vi "Update Zone.vi"(8 "error in (no error)":errorcluster, 9 "Zone Instance":refnum<class "Zone.lvclass">, 10 "Zone Name":string, 11 "TrafficMap in":refnum<class "TrafficMap.lvclass">) -> (0 "error out":errorcluster, 3 "TrafficMap out":refnum<class "TrafficMap.lvclass">)   [LabVIEW 2017, in "TrafficMap.lvclass"]
uses:
  TrafficMap.lvclass
  Zone/Zone.lvclass
  TrafficMap.lvclass/TrafficMap.ctl
  Zone/Zone.lvclass/Zone.ctl
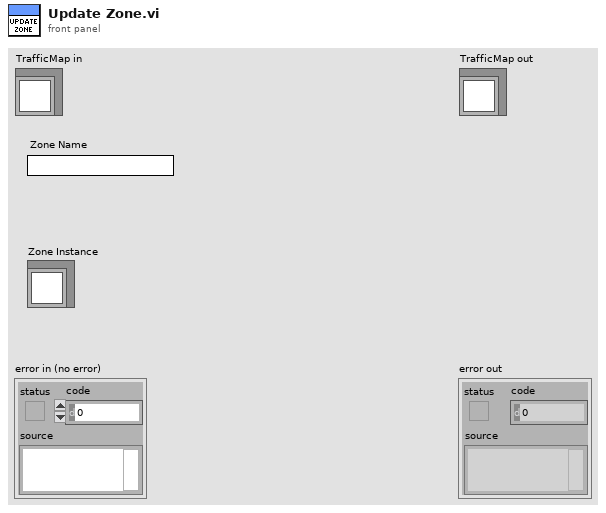
[diagram p1: front panel]
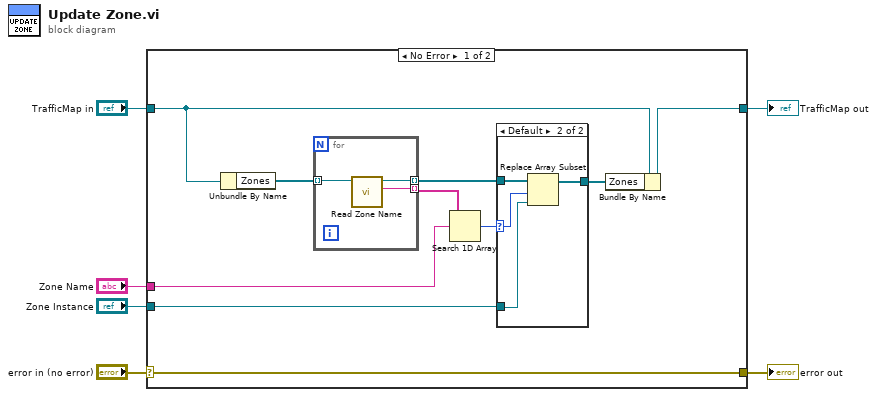
[diagram p0: block diagram]
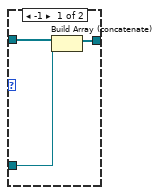
[diagram p2: hidden frame]
diagram:
  n1 = case shown="No Error" "error in (no error)" {
    selector: "error in (no error)" -> [w16 w28]
    tunnel: [w16 w28] -> w5
    tunnel: [w9 w27] -> w3
    tunnel: "TrafficMap in" -> [w10 w27]
    tunnel: "Zone Name" -> [w13 _]
    tunnel: "Zone Instance" -> [w7 _]
    frame No Error {
      n2 = Unbundle By Name(w10) -> ("Zones"=w15:refnum<class "Zone.lvclass">[])
      n3 = for {
        tunnel: w15 -> [w26] mode=indexing
        tunnel: [w25] -> w14 mode=indexing
        tunnel: [w24] -> w11 mode=indexing
        n4 = call "Read Zone Name.vi"("Zone in"=w26) -> ("Zone Name"=w25:string, "Zone out"=w24:refnum<class "Zone.lvclass">)  [unwired: 8 in, 1 out]
      }
      n5 = Search 1D Array(1D array=w14, element=w13) -> (index of element=w12:i32)  [unwired: 1 in]
      n6 = case shown="Default" w12 {
        selector: w12 -> [_ w22]
        tunnel: w11 -> [w17 w23]
        tunnel: [w18 w20] -> w8
        tunnel: w7 -> [w19 w21]
        frame -1 {
          n7 = Build Array (concatenate)(w17, w19) -> (w18:refnum<class "Zone.lvclass">[])
        }
        frame Default {
          n8 = Replace Array Subset(array=w23, new element=w21, index=w22) -> (w20:refnum<class "Zone.lvclass">[])
        }
      }
      n9 = Bundle By Name(cluster=w10, "Zones"=w8) -> (w9:refnum<class "TrafficMap.lvclass">)
    }
    frame Error {
    }
  }
  "error out" <- w5
  "TrafficMap out" <- w3
